vi "set_triggered.vi"(8 "error in (no error)":errorcluster, 10 "triggered?":bool, 11 "DL090202FPGAClock.lvclass in":refnum<class "ClockDL090202FPGA.lvclass">) -> (0 "error out":errorcluster, 3 "DL090202FPGAClock.lvclass out":refnum<class "ClockDL090202FPGA.lvclass">)   [LabVIEW 2010, in "ClockDL090202FPGA.lvclass"]
uses:
  ClockDL090202FPGA.lvclass
  ClockDL090202FPGA.lvclass/ClockDL090202FPGA.ctl
  FPGAWrapper/GenericFPGAWrapper/GenericFPGAWrapper/GenericFPGAWrapper.lvclass
  GenericClock/GenericClock/GenericClock.lvclass
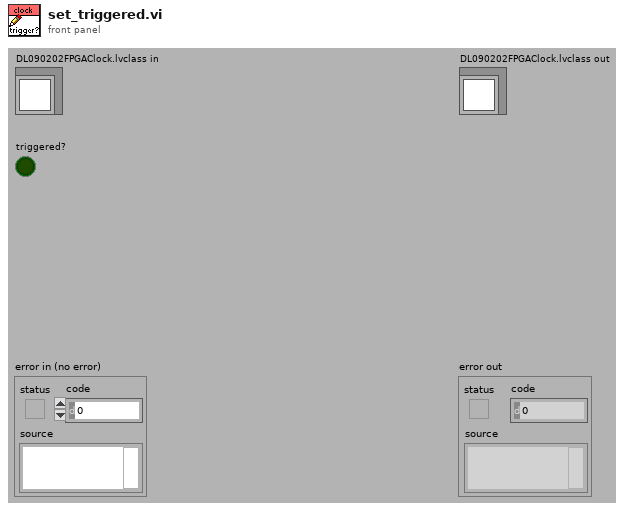
[diagram p1: front panel]
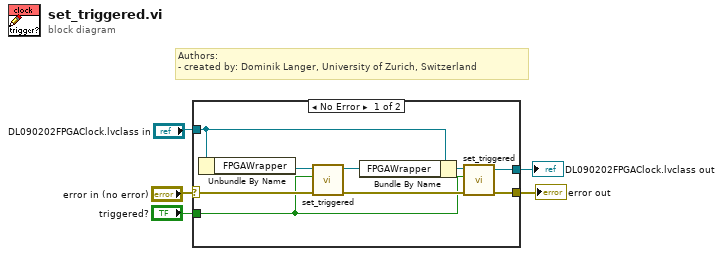
[diagram p0: block diagram]
diagram:
  # "Authors: \n- created by: Dominik Langer, University of Zurich, Switzerland"
  n1 = case shown="No Error" "error in (no error)" {
    selector: "error in (no error)" -> [w13 w15]
    tunnel: [w9 w15] -> w5
    tunnel: "DL090202FPGAClock.lvclass in" -> [w14 w16]
    tunnel: [w7 w16] -> w4
    tunnel: "triggered?" -> [w6 _]
    frame No Error {
      n2 = Unbundle By Name(w14) -> ("FPGAWrapper"=w12:refnum<class "GenericFPGAWrapper.lvclass">)
      n3 = call-dynamic "set_triggered.vi"("error in (no error)"=w13, "triggered?"=w6, "GenericFPGAWrapper in"=w12) -> ("error out"=w10:errorcluster, "GenericFPGAWrapper out"=w11:refnum<class "GenericFPGAWrapper.lvclass">)  [unwired: 7 out]
      n4 = Bundle By Name(cluster=w14, "FPGAWrapper"=w11) -> (w8:refnum<class "ClockDL090202FPGA.lvclass">)
      n5 = call-parent "set_triggered.vi"("error in (no error)"=w10, "triggered?"=w6, "GenericClock.lvclass in"=w8) -> ("error out"=w9:errorcluster, "GenericClock.lvclass out"=w7:refnum<class "ClockDL090202FPGA.lvclass">)  [unwired: 7 out]
    }
    frame Error {
    }
  }
  "error out" <- w5
  "DL090202FPGAClock.lvclass out" <- w4
